vi "Start Stop Scan.vi"(8 "error in (no error)":errorcluster, 10 "Start/Stop":bool, 11 "Generic Data Logger.lvlib:Fluke 2625A (Hydra II).lvlib:Fluke 2625A (Hydra II).lvclass":refnum<class "Fluke 2625A (Hydra II).lvclass">) -> (0 "error out":errorcluster, 3 "Generic Instrument out":refnum<class "Fluke 2625A (Hydra II).lvclass">)   [LabVIEW 2013, in "Generic Data Logger.lvlib" / "Fluke 2625A (Hydra II).lvlib" / "Fluke 2625A (Hydra II).lvclass"]
uses:
  Fluke 2625A (Hydra II).lvclass
  <instrlib>/Fluke 2625A/Fluke 2625A.lvlib
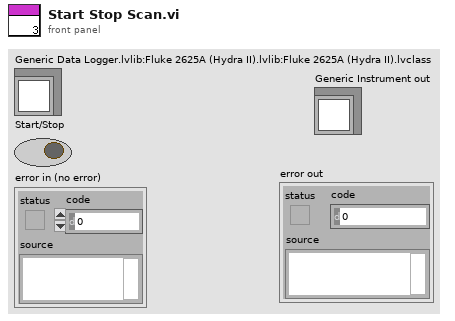
[diagram p1: front panel]
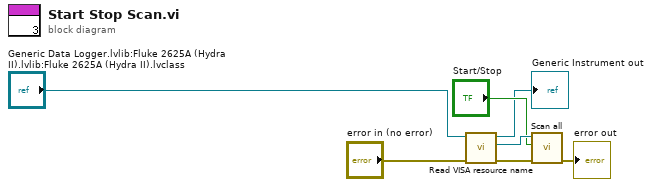
[diagram p0: block diagram]
diagram:
  n1 = call-dynamic "Read VISA resource name.vi"("error in (no error)"="error in (no error)", "Generic Instrument in"="Generic Data Logger.lvlib:Fluke 2625A (Hydra II).lvlib:Fluke 2625A (Hydra II).lvclass") -> ("error out"=w4:errorcluster, "VISA resource name"=w6:refnum<visa-resource-name>, "Generic Instrument out"=→"Generic Instrument out":refnum<class "Fluke 2625A (Hydra II).lvclass">)  [unwired: 7 in]
  n2 = call <instrlib>:"Scan all.vi"("error in (no error)"=w4, "Start/Stop"="Start/Stop", "VISA resource name"=w6) -> ("error out"=→"error out":errorcluster)  [unwired: 7 in, 1 out]
